vi "Loop_Receive From Dashboard.vi"() -> ()   [LabVIEW 2017, in "DashBoardCom.lvlib"]
uses:
  DashBoardCom.lvlib
  Shared Code/TypeDefs/Cluster_DashBoard to Rio Controls.ctl
  Shared Code/TypeDefs/ENUM_Auto Select.ctl
  Global_Dashboard Controls.vi
  Globals/Global_STOP.vi
panel:
  out "Dashboard Controls":T1
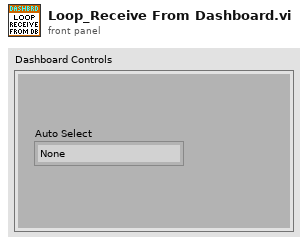
[diagram p1: front panel]
types:
  T1 = typedef "Cluster_DashBoard to Rio Controls.ctl" = cluster{"Auto Select":T2}
  T2 = typedef "ENUM_Auto Select.ctl" = enum16{"None", "Cross Baseline", "Shoot", "Middle Peg", "Right Peg", "Left Peg", "Middle Peg and Shoot", "Side Peg and Shoot", "Dump Hopper and Shoot"}
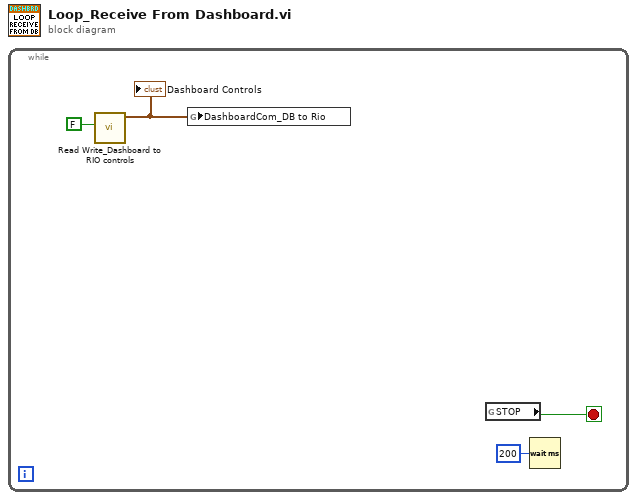
[diagram p0: block diagram]
diagram:
  n1 = while {
    stop <- w3 stop-if-true
    n2 = call "Read Write_Dashboard to RIO controls.vi"("Read(F) Write(T)"=FALSE) -> ("Data Out"=w1:T1)  [unwired: 10 in]
    "Dashboard Controls" <- w1
    n3 = global write "Global_Dashboard Controls.vi" "DashboardCom_DB to Rio"(w1) -> ()
    n4 = global read "Global_STOP.vi" "STOP"() -> (w3:bool)
    n5 = Wait (ms)(milliseconds to wait=u32 200) -> ()  [unwired: 1 out]
  }
